vi "State_Machine.vi"(8 "error in (no error)":errorcluster caption="entrée d'erreur (pas d'erreur)", 11 "Get_Voltage en entrée":refnum<class "Nodon_Set_ZCR_Calibration.lvclass">) -> (0 "error out":errorcluster caption="sortie d'erreur", 2 "Json_String":string, 3 "Get_Voltage en sortie":refnum<class "Nodon_Set_ZCR_Calibration.lvclass">)   [LabVIEW 2020, in "Library Test.lvlib" / "Nodon_Set_ZCR_Calibration.lvclass"]
uses:
  Nodon_Set_ZCR_Calibration.lvclass
  C:/Users/ngarcin/OneDrive - Altyor/Standard TB/Suite TB45/Class/Test/Test (Default)/Test (Default).lvclass
  C:/Users/ngarcin/OneDrive - Altyor/Standard TB/Suite TB45/Class/Test/Nodon_Send_Command_UART/Nodon_Send_Command_UART.lvclass
  Commun VI/TypeDef/Variable Printable.ctl
  JSON API/JSON Value/Set from JSON string.vi
  JSON API/JSON Value/JSON Value.lvclass
  Nodon_Send_Command_UART/Nodon_Send_Command_UART.lvclass
  Commun VI/Library Commun.lvlib
  JSON API/Variant JSON/Variant JSON.lvlib
  JSON API/Get Polymorphic/JSON GetSet.lvlib
  Commun VI/Nodon_ZCR/Nodon_ZCR.lvclass
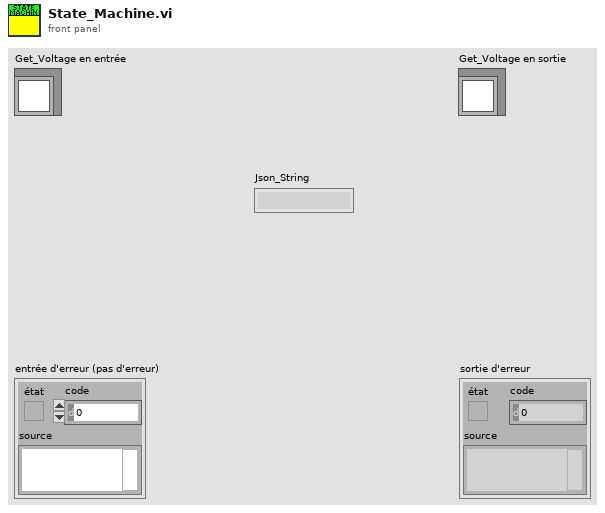
[diagram p1: front panel]
types:
  T1 = typedef "Variable Printable.ctl" = string
  T2 = enum16{"Get Variable", "Get All Variables", "Set Variable", "Delete Variable", "Delete All Variable"}
  T3 = cluster{"Décallage sinus On":dbl, "Décallage sinus Off":dbl}
  T4 = cluster{"Delta relais On (Secondes)":dbl, "Delta relais  Off(Secondes)":dbl}
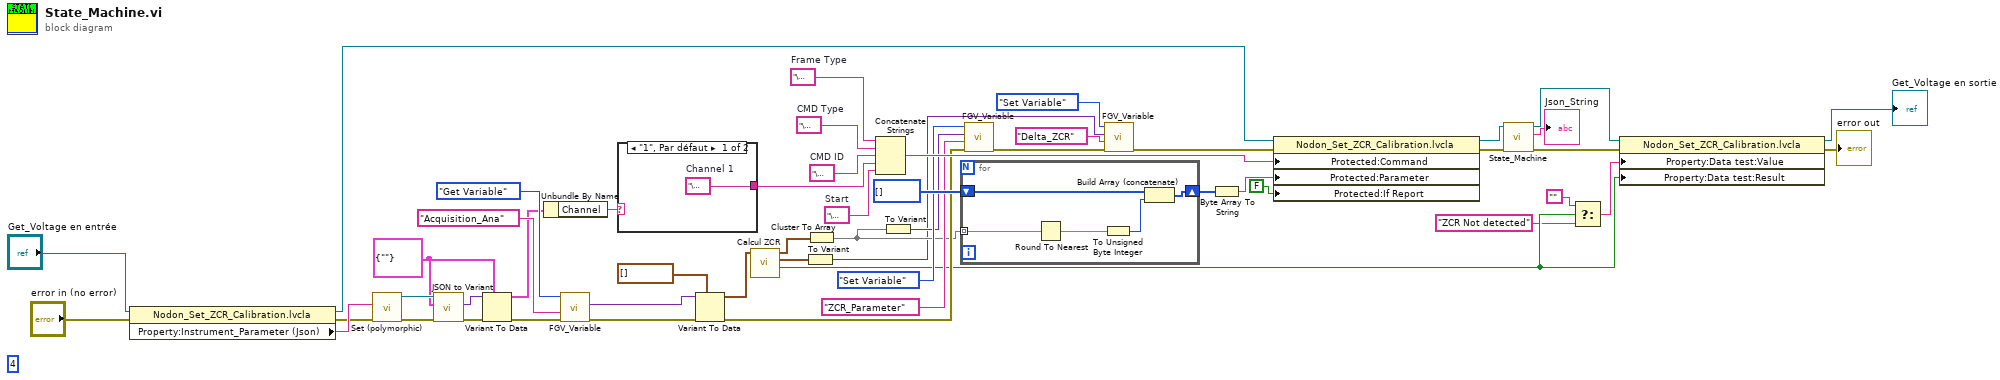
[diagram p0: block diagram]
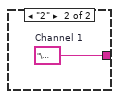
[diagram p2: hidden frame]
diagram:
  (unwired) 4 ("y")
  w30 = cluster{"Channel":string} {"Channel"=""}
  w23 = "\u0000"  # Start
  w49 = "\u0000"  # Frame Type
  w48 = "\u0000"  # CMD ID
  w47 = "\u0003"  # CMD Type
  n1 = property class="Nodon_Set_ZCR_Calibration.lvcla"(reference="Get_Voltage en entrée", error in="error in (no error)") -> (reference out=w22:refnum<class "Nodon_Set_ZCR_Calibration.lvclass">, error out=w31:errorcluster, "Property:Instrument_Parameter (Json)"=w32:string)
  n2 = call-poly "Set (polymorphic).vi"("error in (no error)"=w31, "JSON stream"=w32) -> ("error out"=w34:errorcluster, "JSON Value out"=w36:refnum<class "JSON Value.lvclass">)  [unwired: 7 in, 1 out]
  n3 = call "JSON to Variant.vi"("error in (no error)"=w34, "Variant (Data Type)"=w30, "JSON Value"=w36) -> ("error out"=w35:errorcluster, "Variant out"=w33:variant)  [unwired: 7 in]
  n4 = Variant To Data(error in=w35, type=w30, Variant=w33) -> (data=w29:cluster{"Channel":string}, error out=w26:errorcluster)
  n5 = Unbundle By Name(w29) -> ("Channel"=w25:string)
  n6 = call "FGV_Variable.vi"("error in (no error)"=w26, "Variable"=T1 "Acquisition_Ana", "Function"=T2."Get Variable") -> ("error out"=w42:errorcluster, "Data Out"=w41:variant)  [unwired: 6 in, 1 out]
  n7 = case shown="\"1\", Par défaut" w25 {
    tunnel: [w53 w54] -> w24
    frame "1", Default {
      w53 = "\u0000"  # Channel 1
    }
    frame "2" {
      w54 = "\u0001"  # Channel 1
    }
  }
  n8 = Variant To Data(error in=w42, type=waveform(dbl)[] [] ("data"), Variant=w41) -> (data=w11:waveform(dbl)[], error out=w18:errorcluster)
  n9 = call "Calcul ZCR.vi"("ZCR Signal Input"=w11) -> ("ZCR Valid"=w10:bool, "Controle Decalage"=w3:T3, "Reglage decalage"=w17:T4)  [unwired: 8 in]
  n10 = To Variant(anything=w3) -> (Variant=w4:variant)
  n11 = Cluster To Array(cluster=w17) -> (array=w16:dbl[])
  n12 = Concatenate Strings(w49, w47, w48, w24, w23) -> (w46:string)
  n13 = To Variant(anything=w16) -> (Variant=w19:variant)
  n14 = for {
    shift-right: [w59] -> w38
    shift-left: u8[] [] -> [w58]
    tunnel: w16 -> [w57] mode=indexing
    n15 = Round To Nearest(number=w57) -> (nearest integer value=w55:dbl)
    n16 = To Unsigned Byte Integer(number=w55) -> (unsigned 8bit integer=w56:u8)
    n17 = Build Array (concatenate)(w58, w56) -> (w59:u8[])
  }
  n18 = call "FGV_Variable.vi"("error in (no error)"=w18, "Variable"=T1 "ZCR_Parameter", "Data In"=w19, "Function"=T2."Set Variable") -> ("error out"=w2:errorcluster)  [unwired: 5 in, 2 out]
  n19 = call "FGV_Variable.vi"("error in (no error)"=w2, "Variable"=T1 "Delta_ZCR", "Data In"=w4, "Function"=T2."Set Variable") -> ("error out"=w1:errorcluster)  [unwired: 5 in, 2 out]
  n20 = Byte Array To String(unsigned byte array=w38) -> (string=w37:string)
  n21 = property class="Nodon_Set_ZCR_Calibration.lvcla"(reference=w22, error in=w1, "Protected:Command"=w46, "Protected:Parameter"=w37, "Protected:If Report"=FALSE ("If Report")) -> (reference out=w51:refnum<class "Nodon_Set_ZCR_Calibration.lvclass">, error out=w50:errorcluster)
  n22 = call-parent "State_Machine.vi"("error in (no error)"=w50, "Send_Frame en entrée"=w51) -> ("error out"=w13:errorcluster, "Json_String"=→"Json_String":string, "Send_Frame en sortie"=w15:refnum<class "Nodon_Set_ZCR_Calibration.lvclass">)  [unwired: 7 in]
  n23 = Select(t="", s=w10, f="ZCR Not detected" ("cas faux")) -> (s? t:f=w7:string)
  n24 = property class="Nodon_Set_ZCR_Calibration.lvcla"(reference=w15, error in=w13, "Property:Data test:Value"=w7, "Property:Data test:Result"=w10) -> (reference out=→"Get_Voltage en sortie":refnum<class "Nodon_Set_ZCR_Calibration.lvclass">, error out=→"error out":errorcluster)
